vi "test_13.vi"() -> ()   [LabVIEW 2012]
uses:
  <vilib>/NXT/Dual Mode Library/prims/addArrayElements_int.vi
panel:
  out "center of  'mass'":u16
  in  "array":i16[](array[numeric])
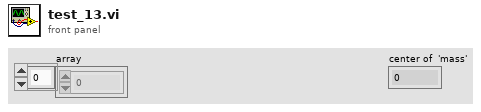
[diagram p1: front panel]
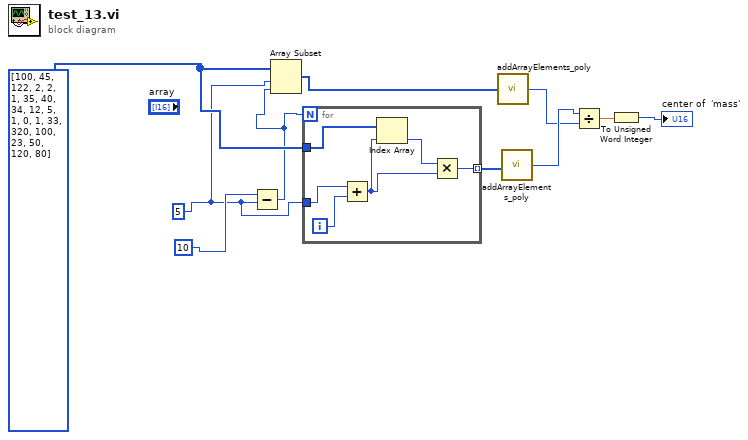
[diagram p0: block diagram]
diagram:
  w2 = 5 ("y")
  w4 = i16[] [100, 45, 122, 2, 2, 1, 35, 40, 34, 12, 5, 1, 0, 1, 33, 320, 100, 23, 50, 120, 80]
  n1 = Subtract(x=10 ("y"), y=w2) -> (x-y=w1:i32)
  n2 = Array Subset(array=w4, index=w2, length=w1) -> (w3:i16[])
  n3 = for {
    N: w1 -> [_]
    tunnel: w2 -> [w15]
    tunnel: w4 -> [w14]
    tunnel: [w11] -> w10 mode=indexing
    i -> [w16]
    n4 = Add(x=w15, y=w16) -> (x+y=w13:i32)
    n5 = Index Array(array=w14, index=w13) -> (element=w12:i16)
    n6 = Multiply(x=w12, y=w13) -> (x*y=w11:i32)
  }
  n7 = call-poly <vilib>:"addArrayElements_poly.vi"("Numeric Array"=w3) -> ("Sum"=w8:i32)
  n8 = call-poly <vilib>:"addArrayElements_poly.vi"("Numeric Array"=w10) -> ("Sum"=w9:i32)
  n9 = Divide(x=w9, y=w8) -> (x/y=w7:dbl)
  n10 = To Unsigned Word Integer(number=w7) -> (unsigned 16bit integer=→"center of  'mass'":u16)
